vi "Configure Acceleration Core.vi"(8 "error in (no error)":errorcluster, 9 "Acceleration":dbl, 10 "AxisNumber":u8, 11 "CS++Nanotec in":refnum<class "CS++Nanotec.lvclass">) -> (0 "error out":errorcluster, 3 "CS++Nanotec out":refnum<class "CS++Nanotec.lvclass">)   [LabVIEW 2015, in "CS++Nanotec.lvlib" / "CS++Nanotec.lvclass"]
doc: "Configures the acceleration (and deceleration) of the axis."
uses:
  CS++Nanotec.lvclass
  CS++Nanotec.lvclass/CS++Nanotec.ctl
  instr.lib/NanotecSMCPD/NanotecSMCPDDriver.lvlib
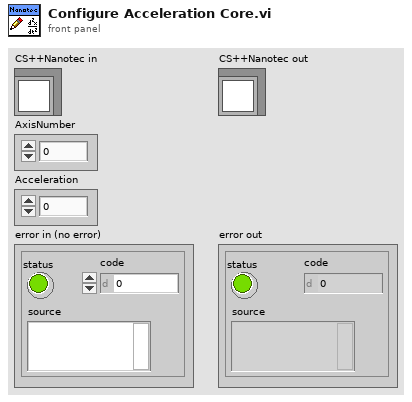
[diagram p1: front panel]
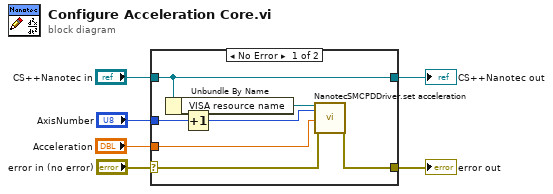
[diagram p0: block diagram]
diagram:
  n1 = case shown="No Error" "error in (no error)" {
    selector: "error in (no error)" -> [w13 w14]
    tunnel: [w12 w14] -> w5
    tunnel: "CS++Nanotec in" -> [w7 w15]
    tunnel: "AxisNumber" -> [w10 _]
    tunnel: "Acceleration" -> [w8 _]
    tunnel: [w7 w15] -> w1
    frame No Error {
      n2 = Unbundle By Name(w7) -> ("VISA resource name"=w11:refnum<visa-resource-name>)
      n3 = Increment(x=w10) -> (x+1=w9:u8)
      n4 = call "NanotecSMCPDDriver.set acceleration.vi"("VISA resource name"=w11, "contollerID"=w9, "acceleration [Hz/s]"=w8, "error in (no error)"=w13) -> ("error out"=w12:errorcluster)  [unwired: 13 in, 2 out]
    }
    frame Error {
    }
  }
  "error out" <- w5
  "CS++Nanotec out" <- w1
